vi "PC Keyboard Control - Defunct.vi"() -> ()   [LabVIEW 2012]
panel:
  out "Rudder":i32
  out "Prop":i32
  out "IR":i32
  in  "stop":bool
  # "Keycodes:\n\nUp = 12\nDown = 13\nLeft = 14\nRight = 15\n\nEnter = 2\nEscape = 22"
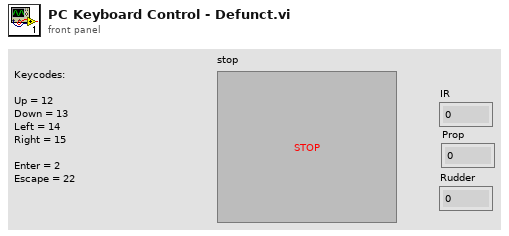
[diagram p1: front panel]
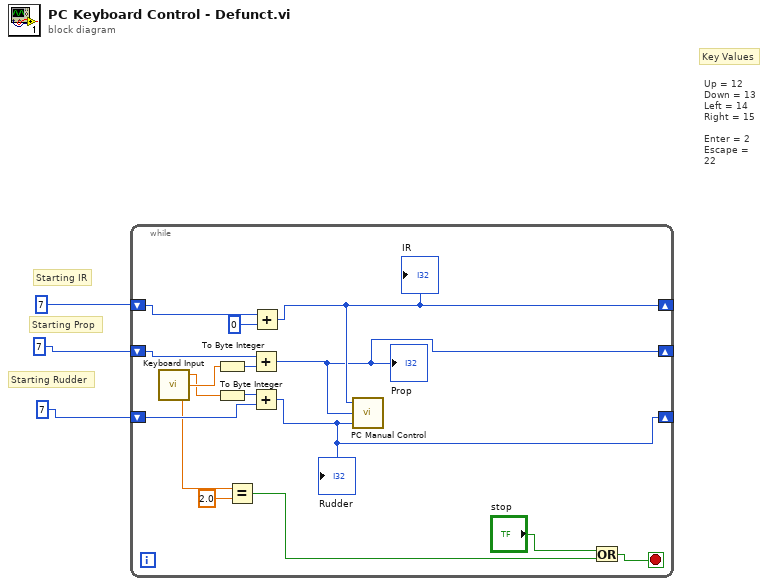
[diagram p0: block diagram]
diagram:
  # "Starting IR"
  # "Starting Prop"
  # "Starting Rudder"
  # "Key Values"
  # "Up = 12\nDown = 13\nLeft = 14\nRight = 15\n\nEnter = 2\nEscape = 22"
  n1 = while {
    shift-right: [w14] -> _
    shift-left: 7 -> [w19]
    shift-right: [w5] -> _
    shift-left: 7 -> [w17]
    shift-right: [w4] -> _
    shift-left: 7 -> [w13]
    stop <- w9 stop-if-true
    n2 = call "Keyboard Input.vi"() -> ("Horizontal Output"=w11:dbl, "Vertical Output"=w15:dbl, "Key Output"=w10:dbl)  [unwired: 2 in]
    n3 = To Byte Integer(number=w15) -> (8bit integer=w16:i8)
    n4 = To Byte Integer(number=w11) -> (8bit integer=w12:i8)
    n5 = Equal?(x=w10, y=2.0) -> (x = y?=w7:bool)
    n6 = Add(x=w17, y=w16) -> (x+y=w5:i32)
    "Prop" <- w5
    n7 = Add(x=w12, y=w13) -> (x+y=w4:i32)
    "Rudder" <- w4
    n8 = Add(x=w19, y=0) -> (x+y=w14:i32)
    "IR" <- w14
    n9 = call "PC Manual Control.vi"("Rudder"=w4, "Prop"=w5, "IR Servo"=w14) -> ()  [unwired: 3 in]
    n10 = Or(x="stop", y=w7) -> (x .or. y?=w9:bool)
  }
